vi "Impedance tube v1.0.3.vi"() -> ()   [LabVIEW 2021]
uses:
  <vilib>/Analysis/1siggen.llb/Ramp Pattern by Samples.vi
  <vilib>/express/express analysis/Spectral/Block/exnSpectralBlock spectral measurements RMS poly.vi
  <vilib>/express/express analysis/Spectral/Block/exnSpectralBlock spectral measurements RMS WFM.vi
  <vilib>/express/express analysis/Spectral/Block/exnSpectralBlock spectral measurements RMS DDT.vi
  <vilib>/Utility/file.llb/Write Delimited Spreadsheet (DBL).vi
  <vilib>/express/express arith-compare/Formula/XNode/ExpressFormulaBlockNode.xnode
  <vilib>/express/express analysis/Spectral/XNode/ExpressSpectralMeasurementsBlockNode.xnode
  <vilib>/Analysis/NI_AALPro.lvlib
  <vilib>/Analysis/NI_AALBase.lvlib
  <vilib>/measure/NI_MABase.lvlib
panel:
  out "freq now1":dbl
  out "Result":i32
  out "Freq now":dbl
  out "fe":dbl
  out "fs":dbl
  out "Dout":cluster{"f0":dbl, "df":dbl, "magnitude":dbl[]}(graph)
  out "Probe":dbl[](graph)
  out "Rr":dbl[](graph)
  out "Absorption coeff":dbl[](graph)
  in  "number of samples":i32=2048
  out "MIC 2":dynamicdata(graph)
  out "MIC 2":dbl
  out "FFT1":dynamicdata(graph)
  out "MIC 1":dynamicdata(graph)
  out "MIC 1":dbl
  in  "stop (F)":bool
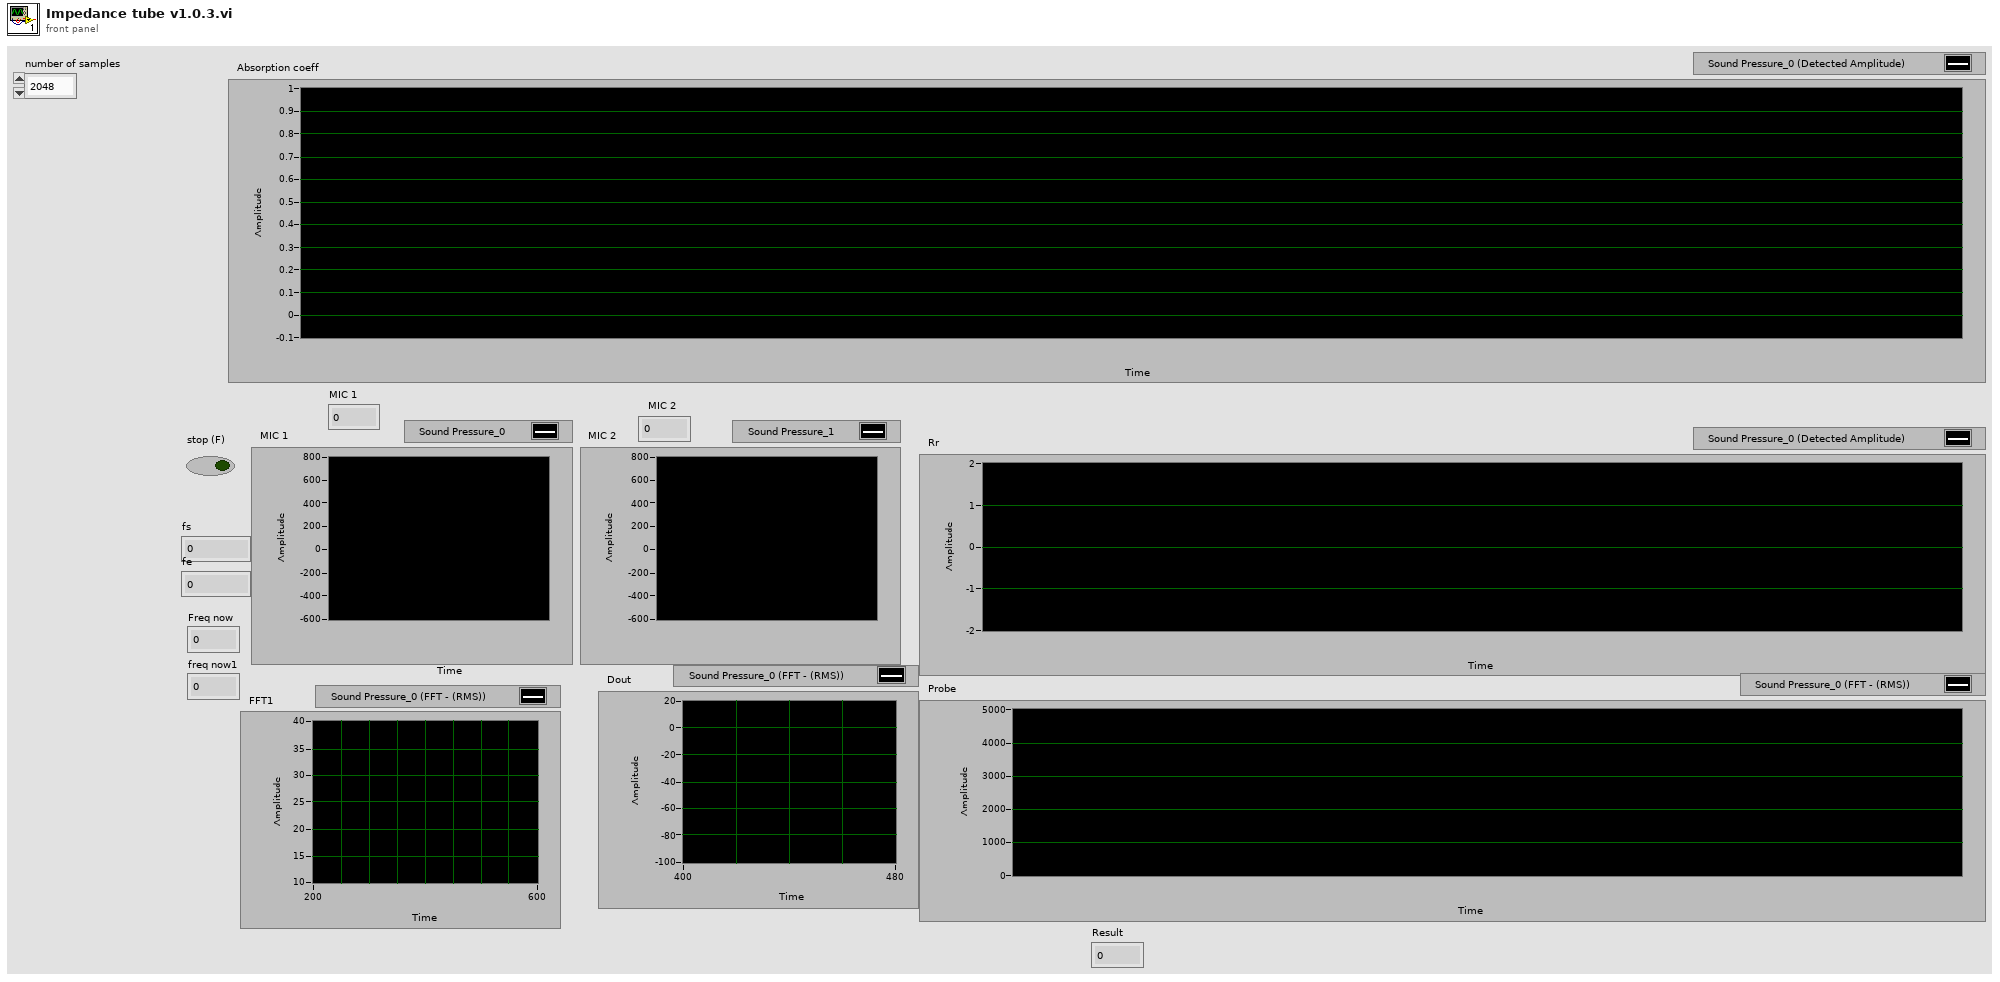
[diagram p1: front panel]
types:
  T1 = cluster{"averaging mode":u16, "weighting mode":u16, "number of averages":u32}
  T2 = cluster{"dB On (F)":bool, "unwrap phase (F)":bool, "convert to degree (F)":bool}
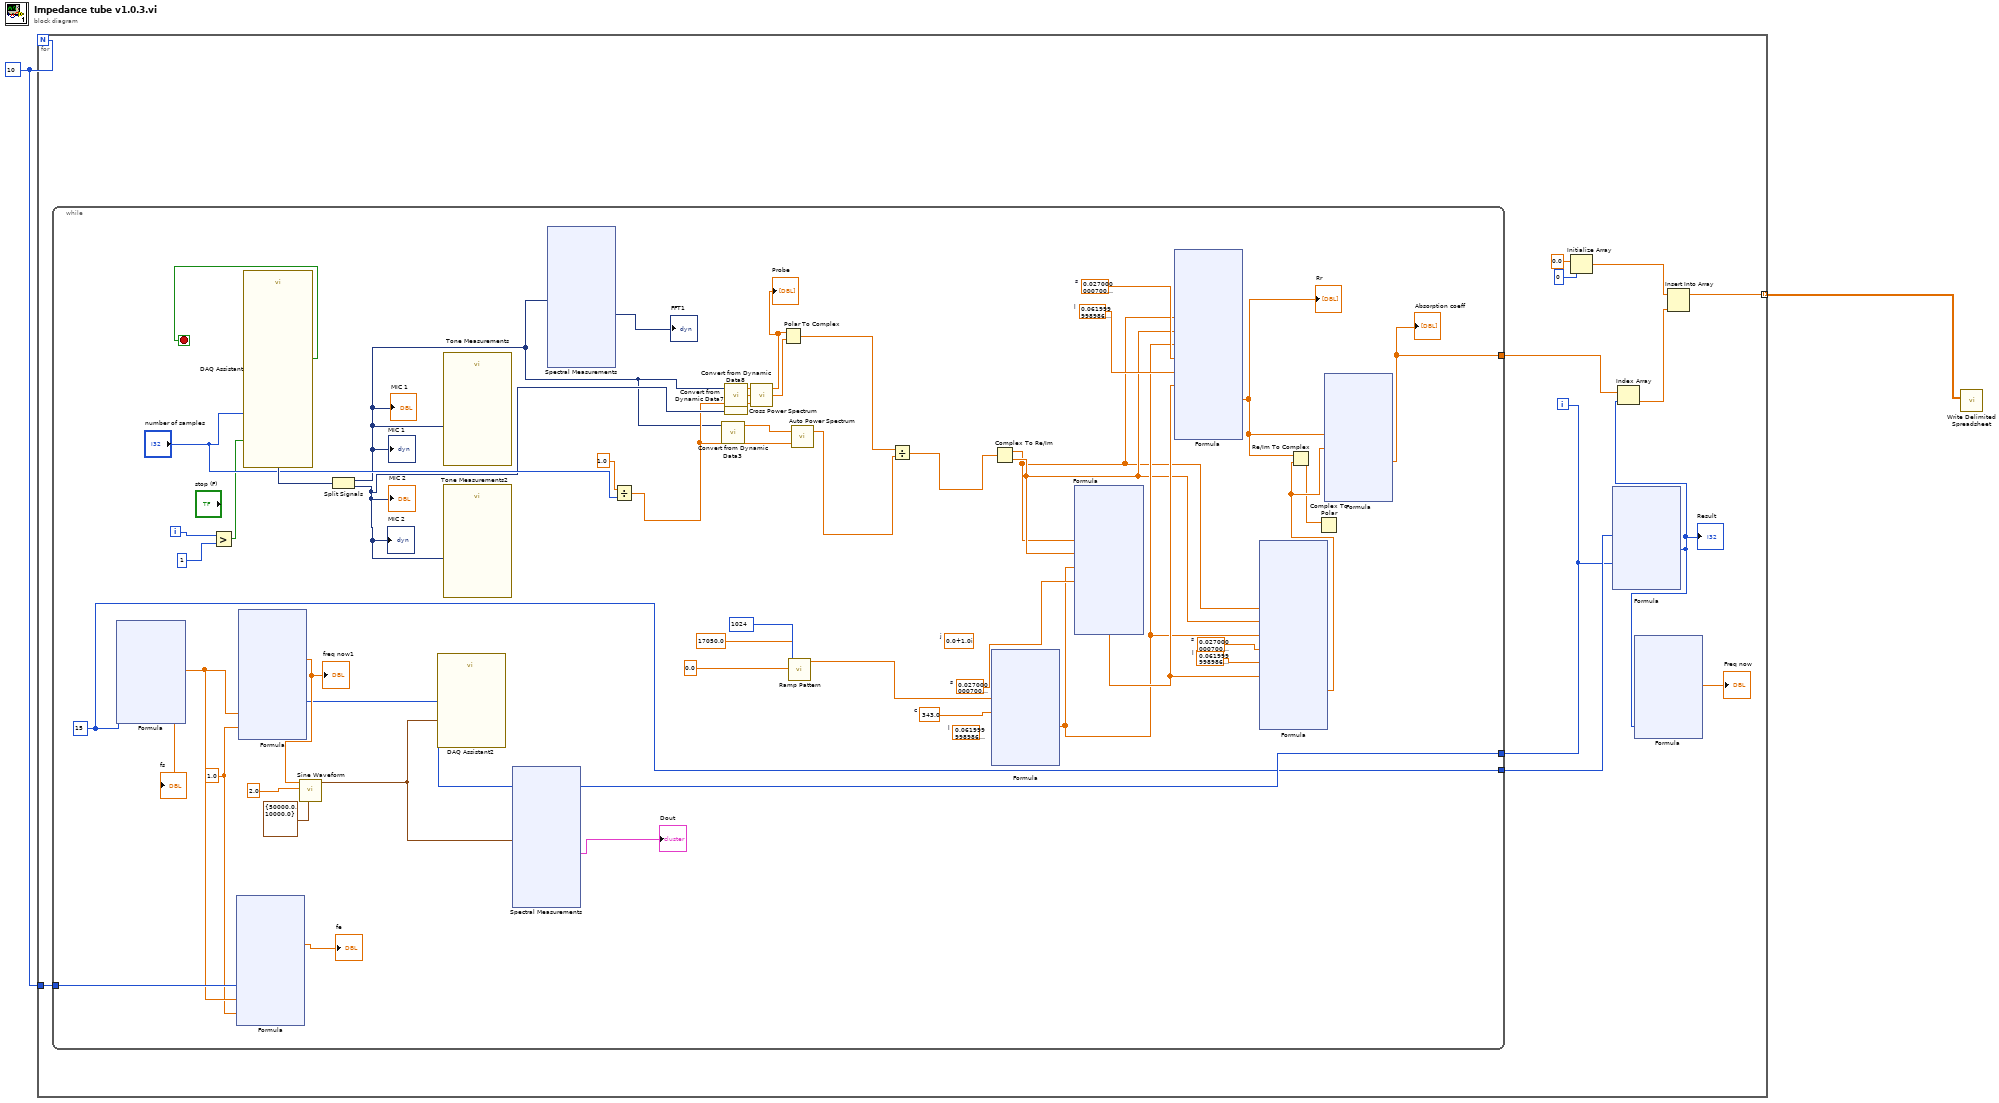
[diagram p0: block diagram]
diagram:
  w1 = 10
  n1 = for {
    N: w1 -> [_]
    tunnel: [w8] -> w2 mode=indexing
    tunnel: w1 -> [w7]
    i -> [w5]
    n2 = while {
      tunnel: [w43] -> w13
      tunnel: w5 -> [w37]
      tunnel: w7 -> [w36]
      tunnel: [w32] -> w6
      i -> [w68]
      stop <- w44 stop-if-true
      w34 = 1.0 ("res")
      w32 = 15 ("n")
      w73 = sgl 0.062  # l
      w74 = sgl 0.027  # s
      w75 = sgl 0.062  # l
      w76 = sgl 0.027  # s
      (unwired) sgl 0.062  # l
      w77 = sgl 0.027  # s
      w78 = sgl 343.0  # c
      (unwired) csg 0.0+1.0i  # j
      n3 = xnode "Formula"("n"=w32) -> ("Result"=w35:dbl)  [unwired: 1 in, 1 out]
      "fs" <- w35
      n4 = Greater?(x=w68, y=1) -> (0:w45:bool)
      n5 = xnode "Formula"("n"=w36, "fs"=w35, "res"=w34) -> ("Result"=→"fe":dbl)  [unwired: 1 in, 1 out]
      n6 = xnode "Formula"("n"=w37, "fs"=w35, "res"=w34) -> ("Result"=w38:dbl)  [unwired: 1 in, 1 out]
      "freq now1" <- w38
      n7 = call "DAQ Assistant"("number of samples"="number of samples", "stop (F)"=w45) -> ("data"=w79:dynamicdata, "stopped"=w44:bool)  [unwired: 14 in, 2 out]
      n8 = call <vilib>:"Sine Waveform.vi"("sampling info"=cluster{"Fs":dbl, "#s":dbl} {"Fs"=50000.0, "#s"=10000.0}, "amplitude"=2.0, "frequency"=w38) -> ("signal out"=w40:waveform(dbl))  [unwired: 7 in, 1 out]
      n9 = Split Signals(w79) -> (w54:dynamicdata, w59:dynamicdata)  [unwired: 2 in]
      "MIC 1" <- w54
      "MIC 1" <- w54
      "MIC 2" <- w59
      "MIC 2" <- w59
      n10 = call "DAQ Assistant2"("data"=w40) -> ()  [unwired: 17 in, 2 out]
      n11 = call "Tone Measurements"("Signals"=w54) -> ()  [unwired: 8 in, 3 out]
      n12 = call "Tone Measurements2"("Signals"=w59) -> ()  [unwired: 8 in, 3 out]
      n13 = xnode "Spectral Measurements"("Signals"=w40) -> ("FFT - (RMS)"=→"Dout":cluster{"f0":dbl, "df":dbl, "magnitude":dbl[]})  [unwired: 1 in, 2 out]
      n14 = xnode "Spectral Measurements"("Signals"=w54) -> ("FFT - (RMS)"=→"FFT1":dynamicdata)  [unwired: 1 in, 2 out]
      n15 = Divide(x=1.0, y="number of samples") -> (x/y=w56:dbl)
      n16 = call "Convert from Dynamic Data3"("Dynamic Data Type"=w54) -> ("Array"=w53:dbl[])  [unwired: 3 in]
      n17 = call "Convert from Dynamic Data7"("Dynamic Data Type"=w54) -> ("Array"=w60:dbl[])  [unwired: 3 in]
      n18 = call "Convert from Dynamic Data8"("Dynamic Data Type"=w59) -> ("Array"=w58:dbl[])  [unwired: 3 in]
      n19 = call <vilib>:"Cross Power Spectrum.vi"("dt"=w56, "Signal Y (V)"=w58, "Signal X (V)"=w60) -> ("Cross Power XY Spectrum Phase (radians)"=w57:dbl[], "Cross Power XY Spectrum Mag (V^2rms)"=w55:dbl[])  [unwired: 1 out]
      "Probe" <- w55
      n20 = Polar To Complex(1:w57, 2:w55) -> (0:w52:cdb[])
      n21 = call-poly <vilib>:"Ramp Pattern.vi"("start"=0.0, "end"=17050.0, "samples"=1024) -> ("Ramp Pattern"=w46:dbl[])  [unwired: 7 in, 1 out]
      n22 = call <vilib>:"Auto Power Spectrum.vi"("dt"=w56, "Signal (V)"=w53) -> ("Power Spectrum (V^2 rms)"=w51:dbl[])  [unwired: 1 out]
      n23 = Divide(x=w52, y=w51) -> (x/y=w50:cdb[])
      n24 = xnode "Formula"("f"=w46, "c"=w78) -> ("Result"=w71:dbl[])  [unwired: 1 in, 1 out]
      n25 = Complex To Re/Im(x + iy=w50) -> (x=w65:dbl[], y=w70:dbl[])
      n26 = xnode "Formula"("Hr"=w65, "Hi"=w70, "k"=w71, "s"=w77) -> ("Result"=w72:dbl[])  [unwired: 1 in, 1 out]
      n27 = xnode "Formula"("Hr"=w65, "Hi"=w70, "k"=w71, "s"=w76, "l"=w75, "D"=w72) -> ("Result"=w62:dbl[])  [unwired: 1 in, 1 out]
      "Rr" <- w62
      n28 = xnode "Formula"("Hr"=w65, "Hi"=w70, "k"=w71, "s"=w74, "l"=w73, "D"=w72) -> ("Result"=w69:dbl[])  [unwired: 1 in, 1 out]
      n29 = Re/Im To Complex(1:w69, 2:w62) -> (0:w66:cdb[])
      n30 = Complex To Polar(r * e^(i*theta)=w66) -> ()  [unwired: 2 out]
      n31 = xnode "Formula"("Rr"=w62, "Ri"=w69) -> ("Result"=w43:dbl[])  [unwired: 1 in, 1 out]
      "Absorption coeff" <- w43
    }
    n32 = Initialize Array(0.0 ("element"), 0 ("dimension size")) -> (w12:dbl[])
    n33 = xnode "Formula"("i1"=w6, "i"=w5) -> ("Result"=w4:i32)  [unwired: 1 in, 1 out]
    "Result" <- w4
    n34 = Index Array(array=w13, index=w4) -> (element=w9:dbl)
    n35 = xnode "Formula"("n"=w4) -> ("Result"=→"Freq now":dbl)  [unwired: 1 in, 1 out]
    n36 = Insert Into Array(array=w12, new element=w9) -> (w8:dbl[])  [unwired: 1 in]
  }
  n37 = call-poly <vilib>:"Write Delimited Spreadsheet.vi"("2D data"=w2) -> ()  [unwired: 13 in, 2 out]
